vi "State3-Found Spot.vi"(10 "Numeric":dbl, 11 "Numeric 2":dbl) -> (1 "Cluster":T2, 2 "Front/Back 2":enum16{"Forward", "Backward", "Stop"}(ring), 3 "Left/Right":enum16{"Left", "Right", "Stop"}(ring), 4 "Enum":T1, 5 "Left/Right Speed":u32)   [LabVIEW 2014]
uses:
  FPGA Bitfiles/Parking States Indicators.ctl
  FPGA Bitfiles/Parking States.ctl
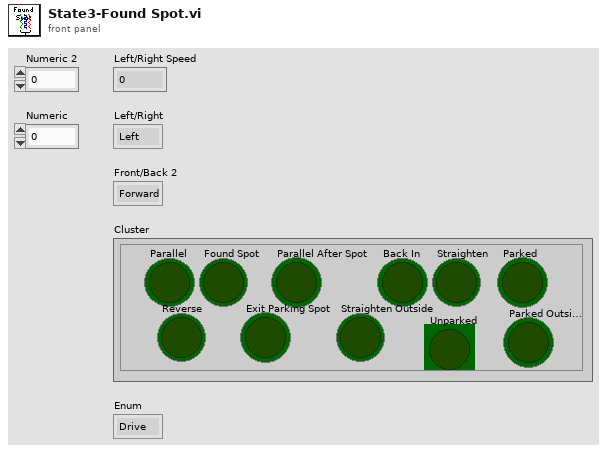
[diagram p1: front panel]
types:
  T1 = typedef "Parking States.ctl" = enum16{"Drive", "Parallel", "Found Spot", "Parallel After Spot", "Back In", "Straighten", "Parked", "Reverse", "Exit Parking Spot", "Straighten Outside", "Unparked", "Parked Outside"}
  T2 = typedef "Parking States Indicators.ctl" = cluster{"Parallel":bool, "Found Spot":bool, "Parallel After Spot":bool, "Back In":bool, "Straighten":bool, "Parked":bool, "Reverse":bool, "Exit Parking Spot":bool, "Straighten Outside":bool, "Unparked":bool, "Parked Outside":bool}
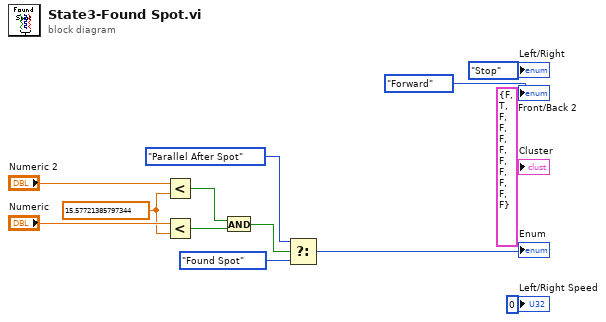
[diagram p0: block diagram]
diagram:
  w4 = 15.57721385797344 ("Distance to detect end of parking spot")
  n1 = Less?(x="Numeric 2", y=w4) -> (x < y?=w1:bool)
  n2 = Less?(x="Numeric", y=w4) -> (x < y?=w2:bool)
  n3 = And(x=w1, y=w2) -> (x .and. y?=w3:bool)
  n4 = Select(t=Parking_States."Parallel After Spot", s=w3, f=Parking_States."Found Spot") -> (s? t:f=→"Enum":T1)
  "Cluster" <- T2 {"Parallel"=FALSE, "Found Spot"=TRUE, "Parallel After Spot"=FALSE, "Back In"=FALSE, "Straighten"=FALSE, "Parked"=FALSE, "Reverse"=FALSE, "Exit Parking Spot"=FALSE, "Straighten Outside"=FALSE, "Unparked"=FALSE, "Parked Outside"=FALSE} ("Cluster")
  "Front/Back 2" <- enum16{"Forward", "Backward", "Stop"}."Forward" ("Front/Back 2")
  "Left/Right" <- enum16{"Left", "Right", "Stop"}."Stop" ("Left/Right")
  "Left/Right Speed" <- u32 0 ("Left/Right Speed")
